vi "BuildTestFromProjectItem_LibraryWithUnsupportedMember_ReturnsError.vi"() -> ()   [LabVIEW 2019, in "LVUnitTestBuilderTest.lvlib"]
uses:
  LVUnitTestBuilderTest.lvlib
  LVUnitTestBuilder/LVUnitTestBuilder.lvclass
  Assertion/Assertion.lvlib
panel:
  out "error out":errorcluster
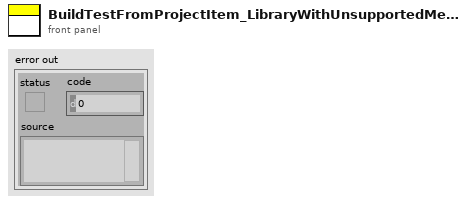
[diagram p1: front panel]
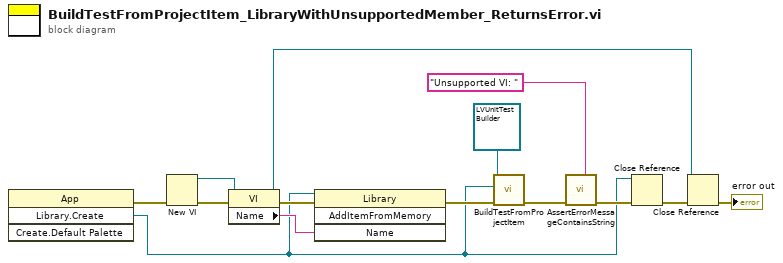
[diagram p0: block diagram]
diagram:
  n1 = invoke class="App" method="Library.Create"() -> (error out=w7:errorcluster, "Create Library"=w4:refnum<vi>)  [unwired: 4 in, 2 out]
  n2 = New VI(8:w7) -> (0:w10:errorcluster, 3:w9:refnum<vi>)  [unwired: 6 in]
  n3 = property class="VI"(reference=w9, error in=w10) -> (reference out=w2:refnum<vi>, error out=w6:errorcluster, "Name"=w8:string)
  n4 = invoke class="Library" method="AddItemFromMemory"(reference=w4, error in=w6, "Name"=w8) -> (error out=w5:errorcluster)  [unwired: 1 in, 3 out]
  n5 = call-dynamic "BuildTestFromProjectItem.vi"("error in (no error)"=w5, "ProjectItem Refnum"=w4, "LVUnitTestBuilder in"=refnum<class "LVUnitTestBuilder.lvclass"> refnum ("LVUnitTestBuilder")) -> ("error out"=w12:errorcluster)  [unwired: 6 in, 2 out]
  n6 = call "AssertErrorMessageContainsString.vi"("Expected"="Unsupported VI: ", "error in (no error)"=w12) -> ("error out"=w11:errorcluster)  [unwired: 9 in]
  n7 = Close Reference(reference=w4, error in (no error)=w11) -> (error out=w13:errorcluster)
  n8 = Close Reference(reference=w2, error in (no error)=w13) -> (error out=→"error out":errorcluster)
